vi "Result View.vi"(8 "error in (no error)":errorcluster, 11 "Coverage Report In":refnum<class "Coverage Report.lvclass">) -> (0 "error out":errorcluster, 3 "Coverage Report Out":refnum<class "Coverage Report.lvclass">)   [LabVIEW 2020, in "Coverage Report.lvclass"]
uses:
  Coverage Report.lvclass
  Coverage Report.lvclass/Coverage Report.ctl
  <vilib>/Analysis/baseanly.llb/Mean (DBL).vi
  <vilib>/Analysis/NI_AALBase.lvlib
panel:
  in  "VI tree":string[](tree)
  out "Summary":string
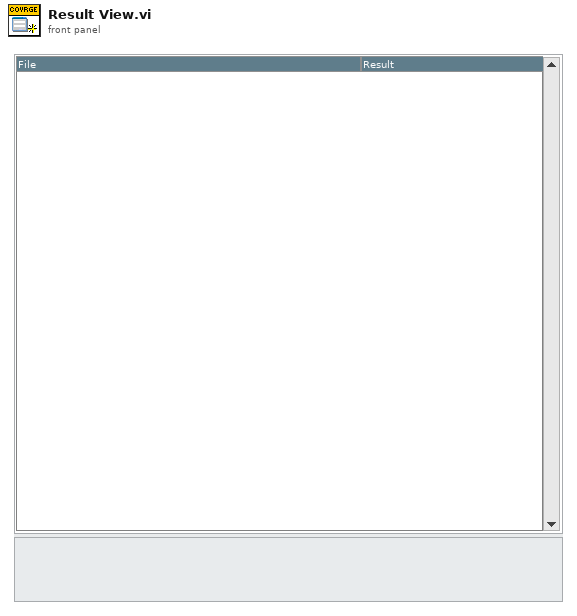
[diagram p1: front panel]
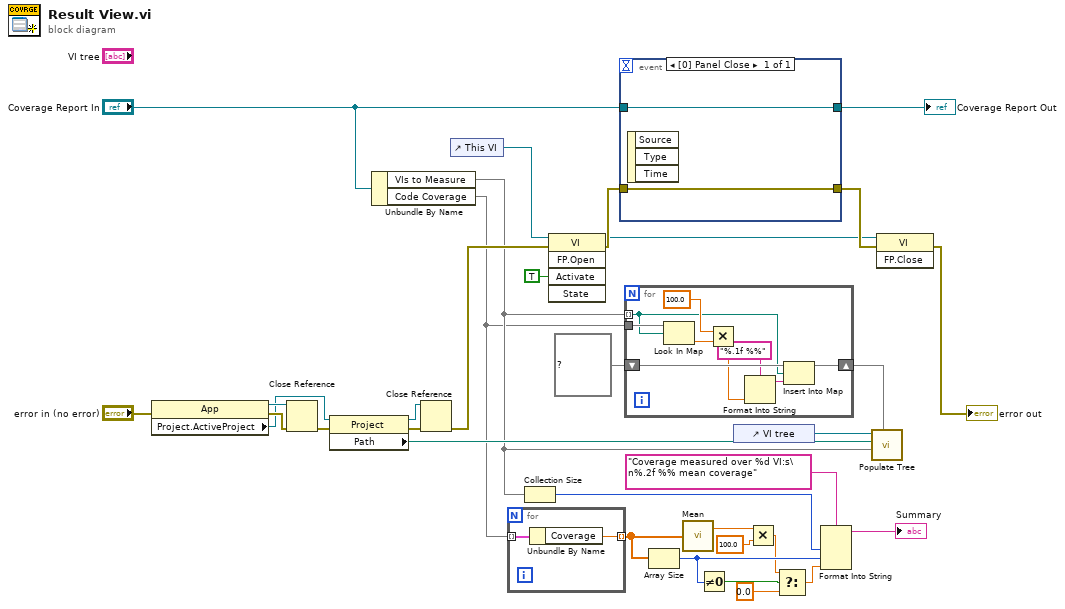
[diagram p0: block diagram]
diagram:
  n1 = property class="App"(error in="error in (no error)") -> (reference out=w21:refnum<vi>, error out=w24:errorcluster, "Project.ActiveProject"=w20:refnum<vi>)  [unwired: 1 in]
  n2 = Close Reference(reference=w21, error in (no error)=w24) -> (error out=w25:errorcluster)
  n3 = property class="Project"(reference=w20, error in=w25) -> (reference out=w22:refnum<vi>, error out=w23:errorcluster, "Path"=w19:path)
  n4 = Unbundle By Name("Coverage Report In") -> ("VIs to Measure"=w13:set{path}, "Code Coverage"=w12:map{path, dbl})
  n5 = Close Reference(reference=w22, error in (no error)=w23) -> (error out=w17:errorcluster)
  n6 = control-ref of="This VI"() -> (w26:refnum<vi>)
  n7 = for {
    tunnel: [w34] -> w11 mode=indexing
    tunnel: w12 -> [w35] mode=indexing
    n8 = Unbundle By Name(w35) -> ("Coverage"=w34:dbl)
  }
  n9 = Collection Size(1:w13) -> (0:w9:i32)
  n10 = invoke class="VI" method="FP.Open"(reference=w26, error in=w17, "Activate"=TRUE ("Activate?")) -> (reference out=w14:refnum<vi>, error out=w28:errorcluster)  [unwired: 2 in, 3 out]
  n11 = event shown="[0] Panel Close" {
    selector: _ -> [_]
    dyn-events: _ -> [_]
    timeout: _ -> [_]
    tunnel: w28 -> [w37]
    tunnel: [w37] -> w27
    tunnel: "Coverage Report In" -> [w36]
    tunnel: [w36] -> w15
    event Panel Close {
      n12 = event-data() -> ()  [unwired: 1 in, 3 out]
    }
  }
  "Coverage Report Out" <- w15
  n13 = for {
    tunnel: w13 -> [w40] mode=indexing
    shift-right: [w44] -> w31
    shift-left: map{path, string} {} ("Results") -> [w46]
    tunnel: w12 -> [w45]
    n14 = Look In Map(map=w45, key=w40) -> (value=w43:dbl)  [unwired: 1 in, 1 out]
    n15 = Multiply(x=100.0, y=w43) -> (x*y=w38:dbl)
    n16 = Format Into String(format string="%.1f %%", w38) -> (resulting string=w41:string)  [unwired: 2 in, 1 out]
    n17 = Insert Into Map(map in=w46, key=w40, value=w41) -> (map out=w44:map{path, string})  [unwired: 2 out]
  }
  n18 = Array Size(array=w11) -> (size(s)=w7:i32)
  n19 = call-poly <vilib>:"Mean.vi"("X"=w11) -> ("mean"=w5:dbl)  [unwired: 1 out]
  n20 = Not Equal To 0?(x=w7) -> (x != 0?=w6:bool)
  n21 = control-ref of="VI tree"() -> (w33:refnum<vi>)
  n22 = Multiply(x=w5, y=100.0) -> (x*y=w2:dbl)
  n23 = Select(t=w2, s=w6, f=0.0) -> (s? t:f=w3:dbl)
  n24 = Format Into String(format string="Coverage measured over %d VI:s\n%.2f %% mean coverage", w9, w7, w3) -> (resulting string=→"Summary":string)  [unwired: 2 in, 1 out]
  n25 = call "Populate Tree.vi"("Results"=w31, "VIs"=w13, "Project Path"=w19, "TreeControl in"=w33) -> ()  [unwired: 7 in, 1 out]
  n26 = invoke class="VI" method="FP.Close"(reference=w14, error in=w27) -> (error out=→"error out":errorcluster)  [unwired: 1 in, 2 out]
